vi "lab1.vi"() -> ()   [LabVIEW 2020]
uses:
  <vilib>/measure/NI_MABase.lvlib
panel:
  out "Numérique":i32
  out "données":dbl
  out "data":dynamicdata(graph) caption="données"
  in  "stop (F)":bool
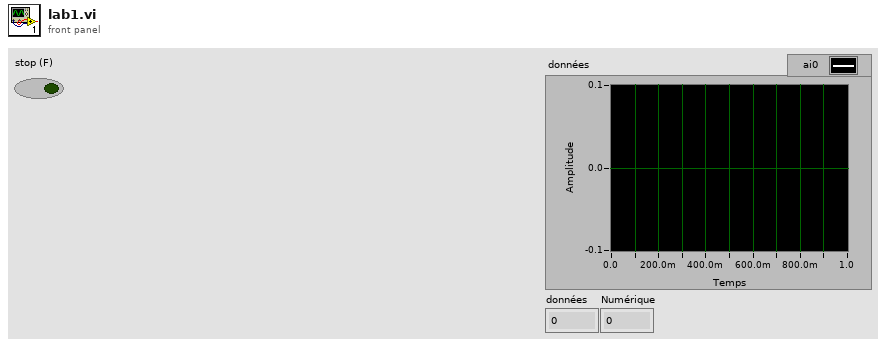
[diagram p1: front panel]
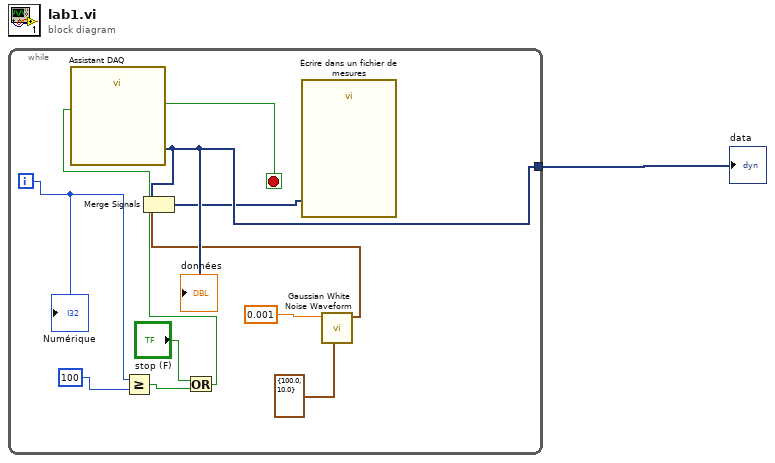
[diagram p0: block diagram]
diagram:
  n1 = while {
    tunnel: [w11] -> w1
    i -> [w10]
    stop <- w12 stop-if-true
    n2 = Greater Or Equal?(x=w10, y=100) -> (x >= y?=w8:bool)
    n3 = Or(x="stop (F)", y=w8) -> (x .or. y?=w6:bool)
    n4 = call "Assistant DAQ"("stop (F)"=w6) -> ("data"=w11:dynamicdata, "stopped"=w12:bool)  [unwired: 15 in, 2 out]
    "données" <- w11
    n5 = call <vilib>:"Gaussian White Noise Waveform.vi"("sampling info"=cluster{"Fs":dbl, "#s":dbl} {"Fs"=100.0, "#s"=10.0}, "standard deviation"=0.001) -> ("signal out"=w2:waveform(dbl))  [unwired: 8 in, 1 out]
    n6 = Merge Signals(w11, w2) -> (w3:dynamicdata)
    n7 = call "Écrire dans un fichier de mesures"("Signals"=w3) -> ()  [unwired: 16 in, 3 out]
    "Numérique" <- w10
  }
  "data" <- w1
